vi "Acquisition Message Loop.vi"(8 "error in (no error)":errorcluster, 9 "data queue in":refnum<queue>, 10 "notifier out":refnum<notifier>, 11 "Message Queues":T3) -> (0 "error out":errorcluster)   [LabVIEW 2026, in "Acquisition.lvlib"]
doc: "Message loop for handling messages pertaining to the acquisition of data from the hardware."
uses:
  Acquisition.lvlib
  support/Message Queue/All Message Queues.ctl
  support/Message Queue/Message Cluster.ctl
  controls/NotifierAndDataQueue.ctl
  controls/WaveformChartData.ctl
  Hardware Configuration.ctl
  Acquisition State.ctl
  support/Message Queue/Enqueue Message (Single).vi
  <vilib>/Utility/error.llb/Error Cluster From Error Code.vi
  <vilib>/ErrorRing/Error Ring.xnode
  support/Message Queue/Message Queue.lvlib
  <vilib>/Utility/miscctls.llb/LVRowAndColumnTypeDef.ctl
  Control/Control.lvlib
  Settings/Settings.lvlib
panel:
  out "STOP Button Pressed 4":bool
  out "Pressure Decay Hold Test Complete":bool
  out "STOP Button Pressed 3":bool
  out "Timeout":bool
  out "Pressure Stabilized":bool
  out "STOP Button Pressed 2":bool
  out "Free Air Flow Measurement Complete":bool
  out "RPM Target Reached":bool
  out "STOP Button Pressed":bool
  out "RPM Timeout":bool
  in  "Notifier Data":T1
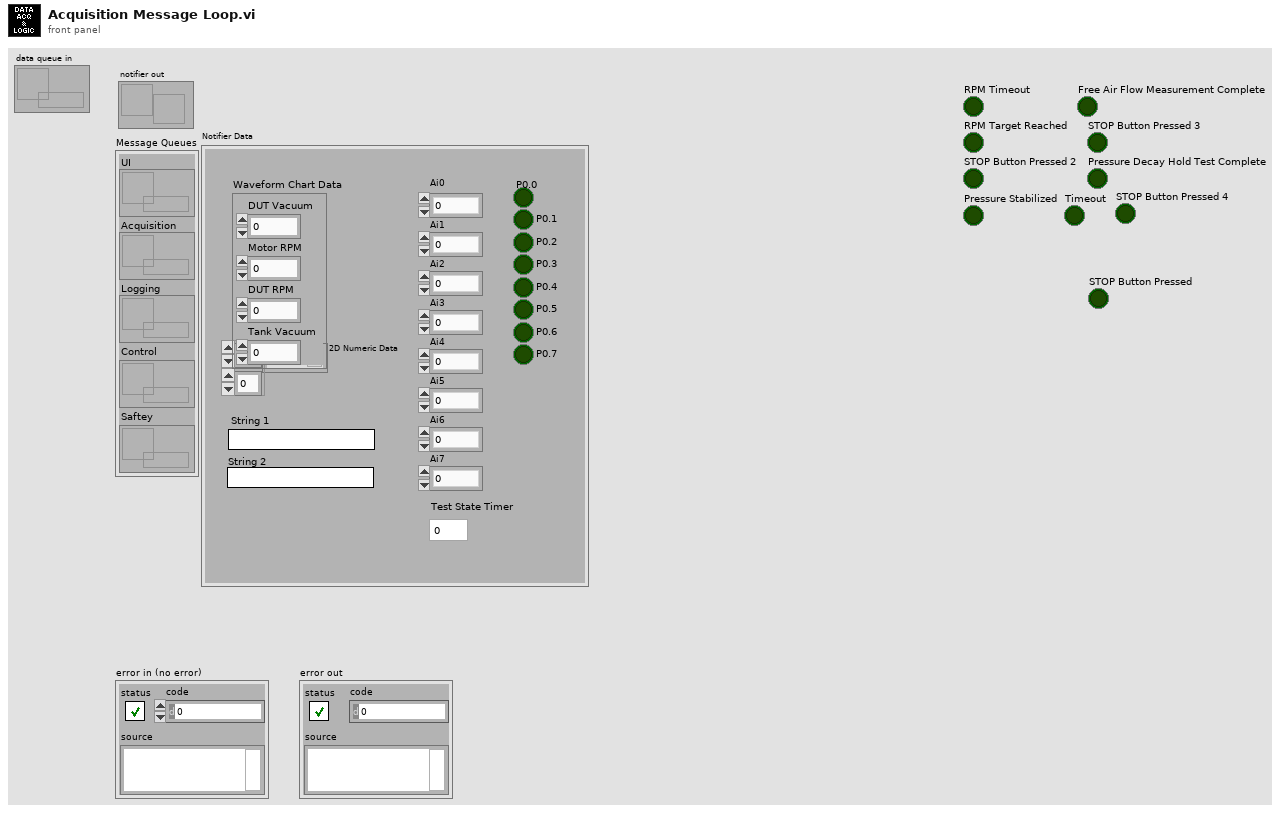
[diagram p1: front panel]
types:
  T1 = typedef "NotifierAndDataQueue.ctl" = cluster{"Ai0":dbl, "Ai1":dbl, "Ai2":dbl, "Ai3":dbl, "Ai4":dbl, "Ai5":dbl, "Ai6":dbl, "Ai7":dbl, "P0.0":bool, "P0.1":bool, "P0.2":bool, "P0.3":bool, "P0.4":bool, "P0.5":bool, "P0.6":bool, "P0.7":bool, "2D Numeric Data":dbl[][], "String 2":string, "String 1":string, "Waveform Chart Data":T2, "Test State Timer":dbl}
  T2 = typedef "Settings.lvlib/WaveformChartData.ctl" = cluster{"DUT Vacuum":dbl, "Motor RPM":dbl, "DUT RPM":dbl, "Tank Vacuum":dbl}
  T3 = typedef "Message Queue.lvlib/All Message Queues.ctl" = cluster{"UI":refnum<queue>, "Acquisition":refnum<queue>, "Logging":refnum<queue>, "Control":refnum<queue>, "Saftey":refnum<queue>}
  T4 = typedef "Acquisition.lvlib/Acquisition State.ctl" = enum16{"Idle", "Acquiring"}
  T5 = typedef "Acquisition.lvlib/Hardware Configuration.ctl" = cluster{"Analog Out array":dbl[], "Initialize Flag":bool, "Saftey Table Display":refnum<vi>, "Torque&Force":waveform(dbl)[][], "Calibration Data":waveform(dbl)[], "2D":dbl[][], "Analog In Task":refnum<k21>, "Digital In Task":refnum<k21>, "Analog Out Task":refnum<k21>, "Digital Out Task":refnum<k21>, "Digital Out Array":bool[], "Current Cycle Count":refnum<vi>, "Cycle Count":u64, "Headers":string[], "Sweep Interval":u64, "Delay":u64, "TestConfigDisplay":refnum<vi>, "50psi Conversion":dbl[], "1245N15 Conversion":dbl[], "MX06F Conversion":dbl[], "# of Test Cycles":u64, "60psi Conversion":dbl[], "100psi Conversion":dbl[], "200psi Conversion":dbl[], "1000psi Conversion":dbl[], "2000psi Conversion":dbl[], "5000psi Conversion":dbl[], "MX09F Conversion":dbl[], "MX19F Conversion":dbl[], "DUT VALVE POSITION":refnum<vi>, "INTAKE VALVE POSITION":refnum<vi>, "Table Control":refnum<vi>, "Table Control":string[][], "Max Vacuum":dbl, "RPM Ramp Ref":refnum<vi>, "Free Air Flow Ref":refnum<vi>, "Press Stable Ref":refnum<vi>, "Press Decay Ref":refnum<vi>}
  T6 = typedef "LVRowAndColumnTypeDef.ctl" = cluster{"Row":i32, "Column":i32}
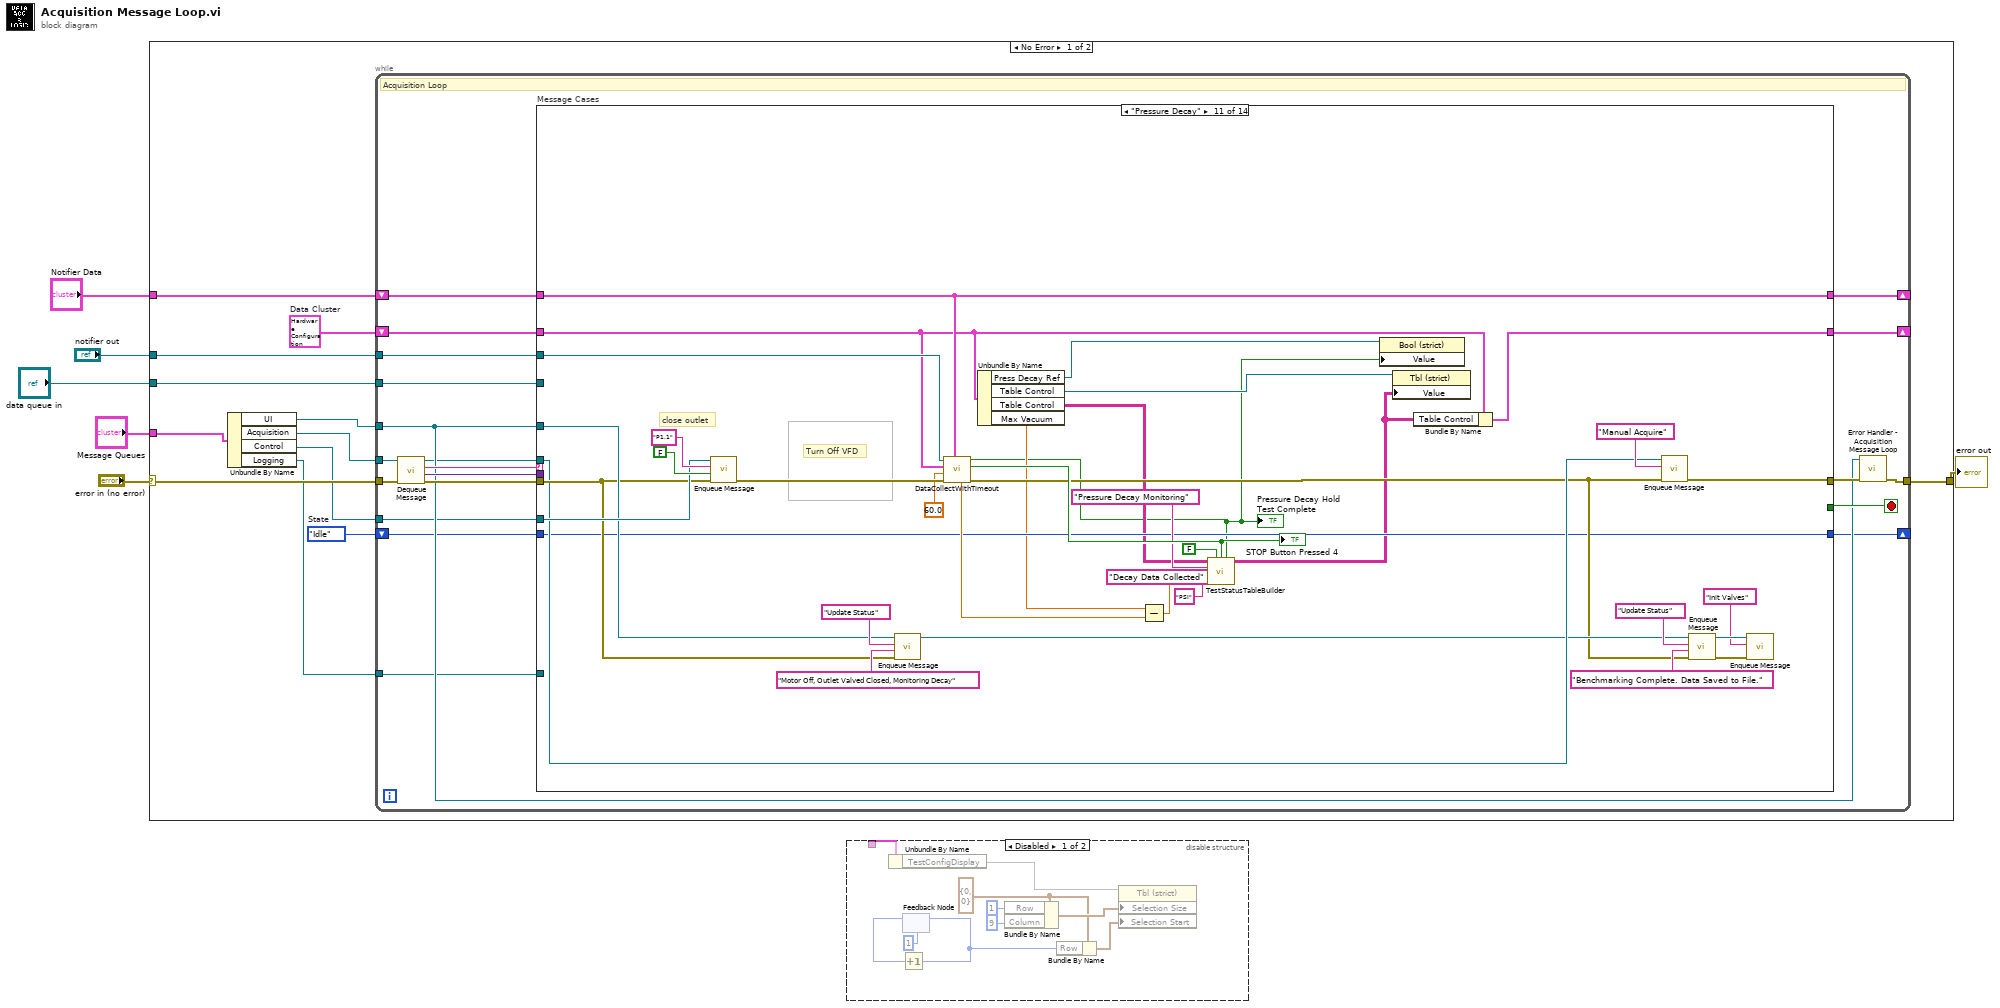
[diagram p0: block diagram]
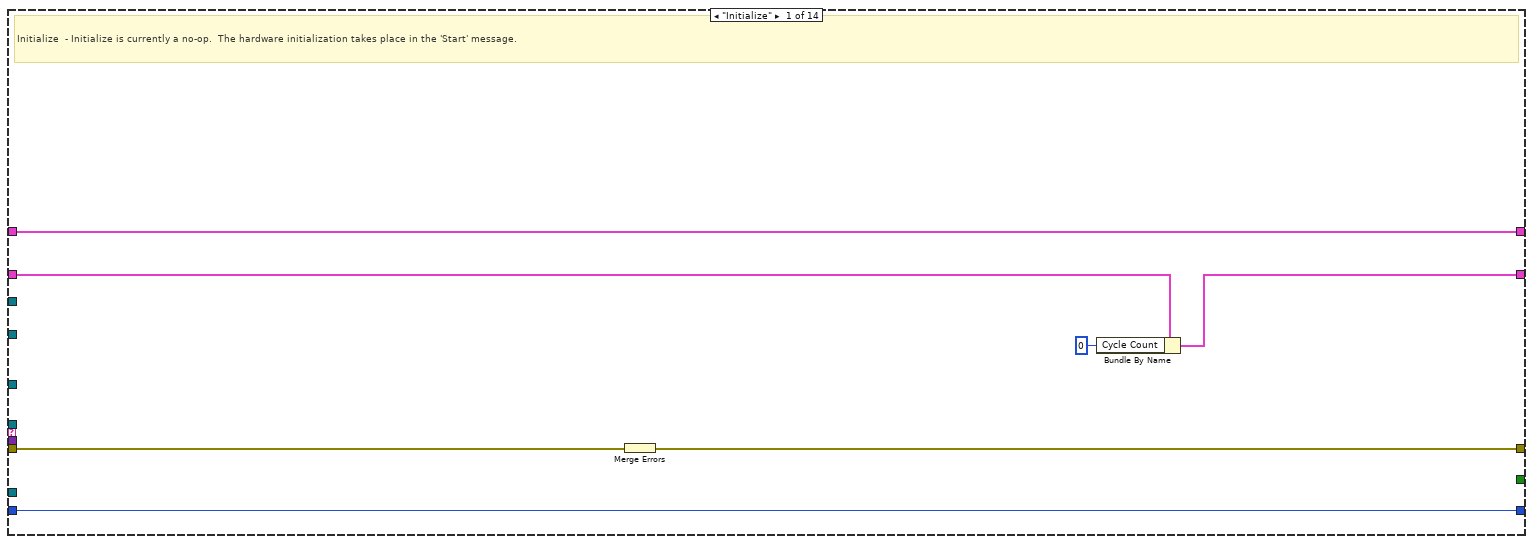
[diagram p3: hidden frame]
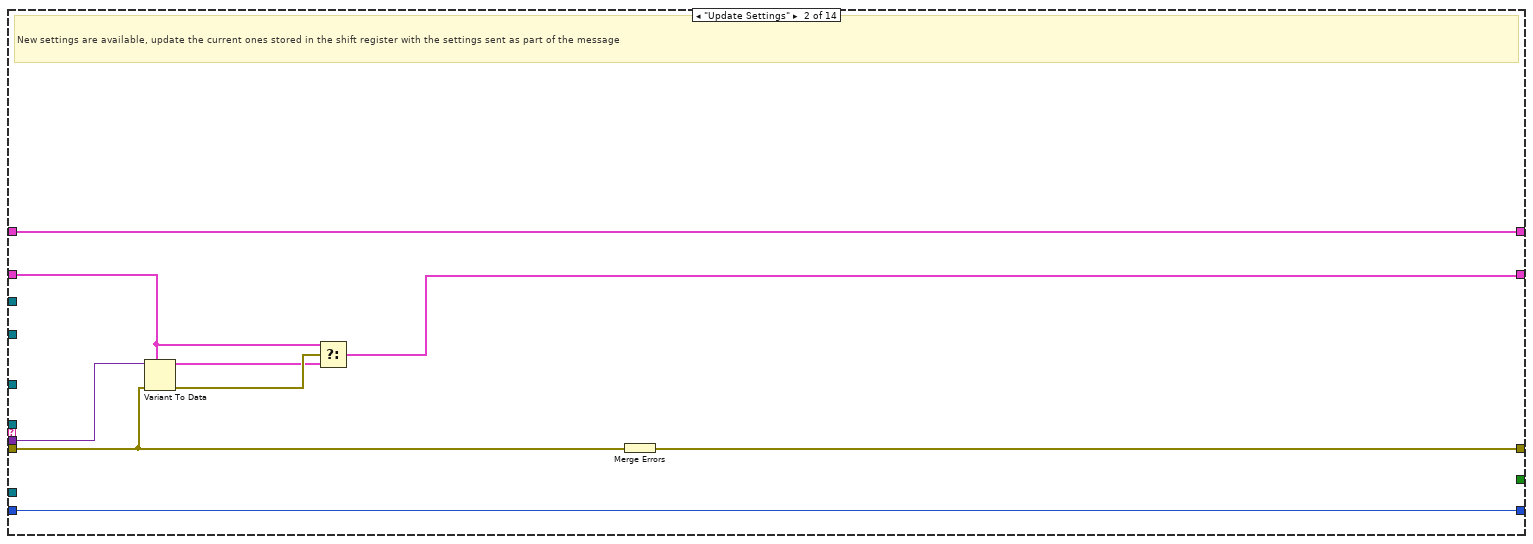
[diagram p4: hidden frame]
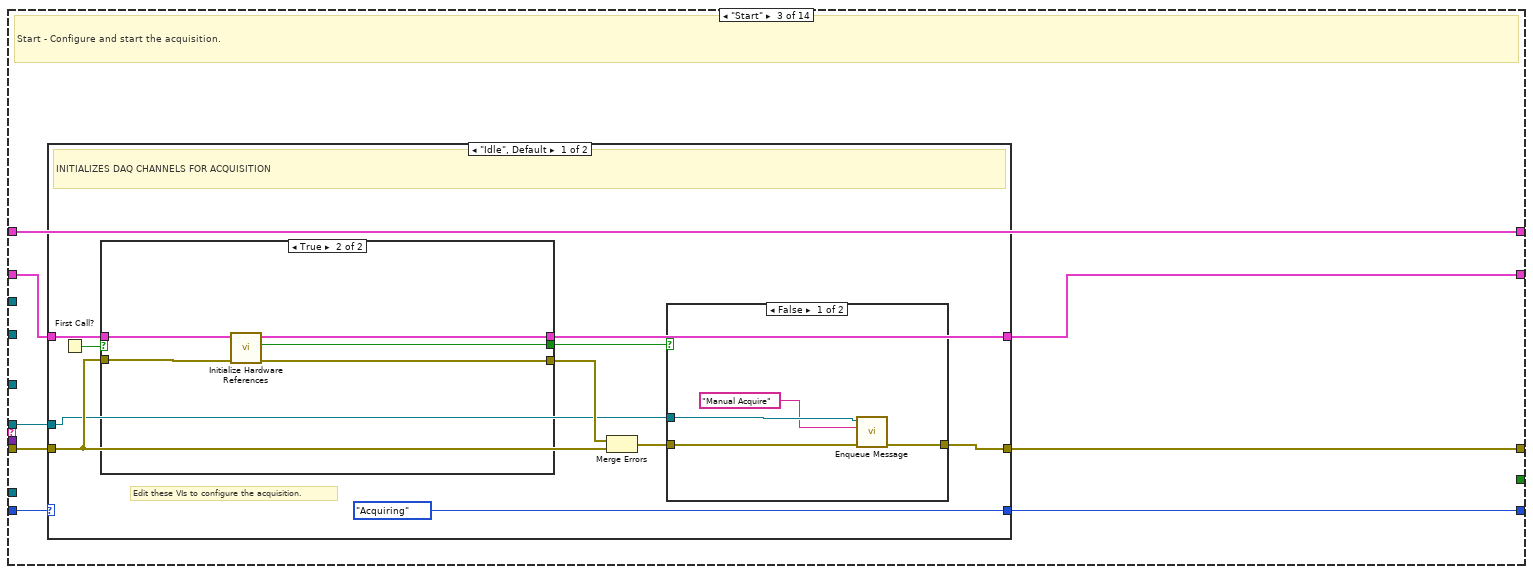
[diagram p5: hidden frame]
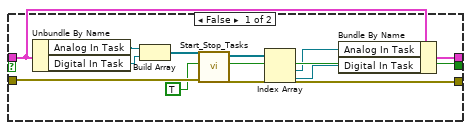
[diagram p6: hidden frame]
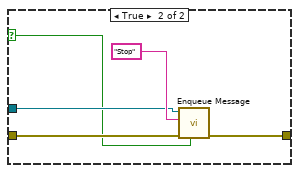
[diagram p7: hidden frame]
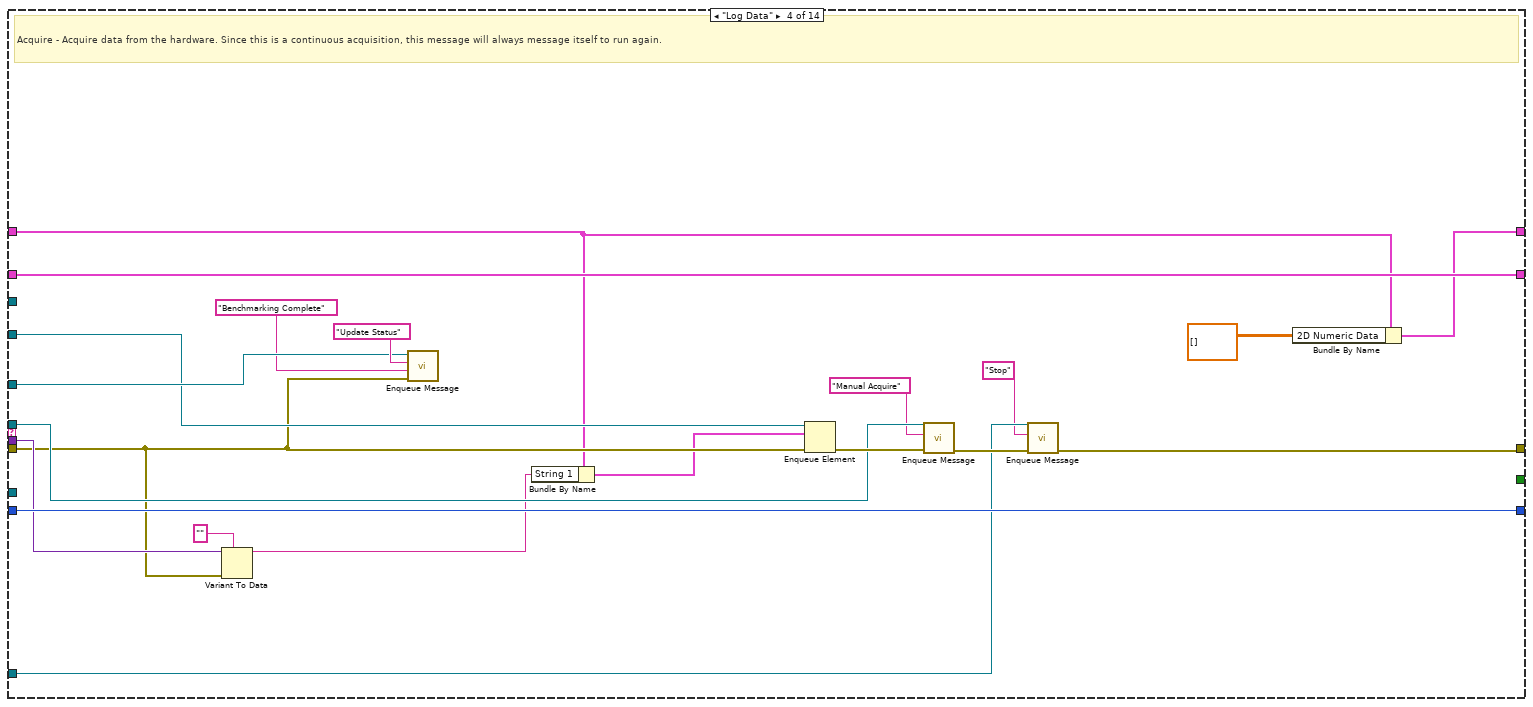
[diagram p9: hidden frame]
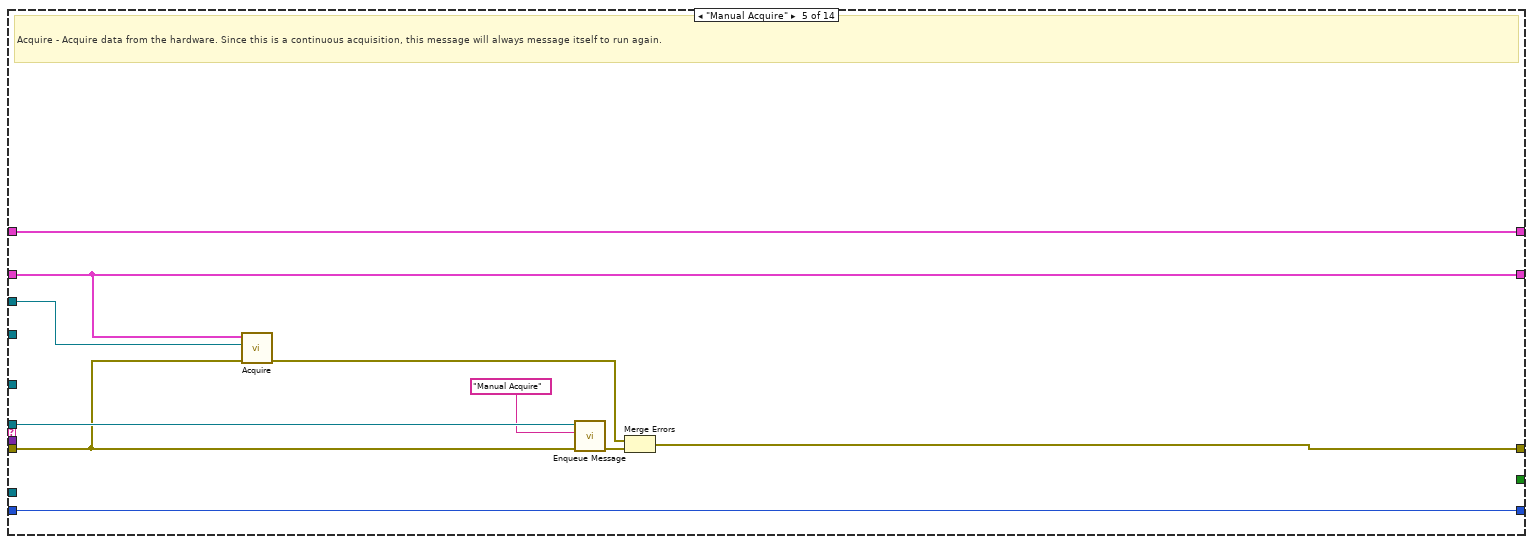
[diagram p10: hidden frame]
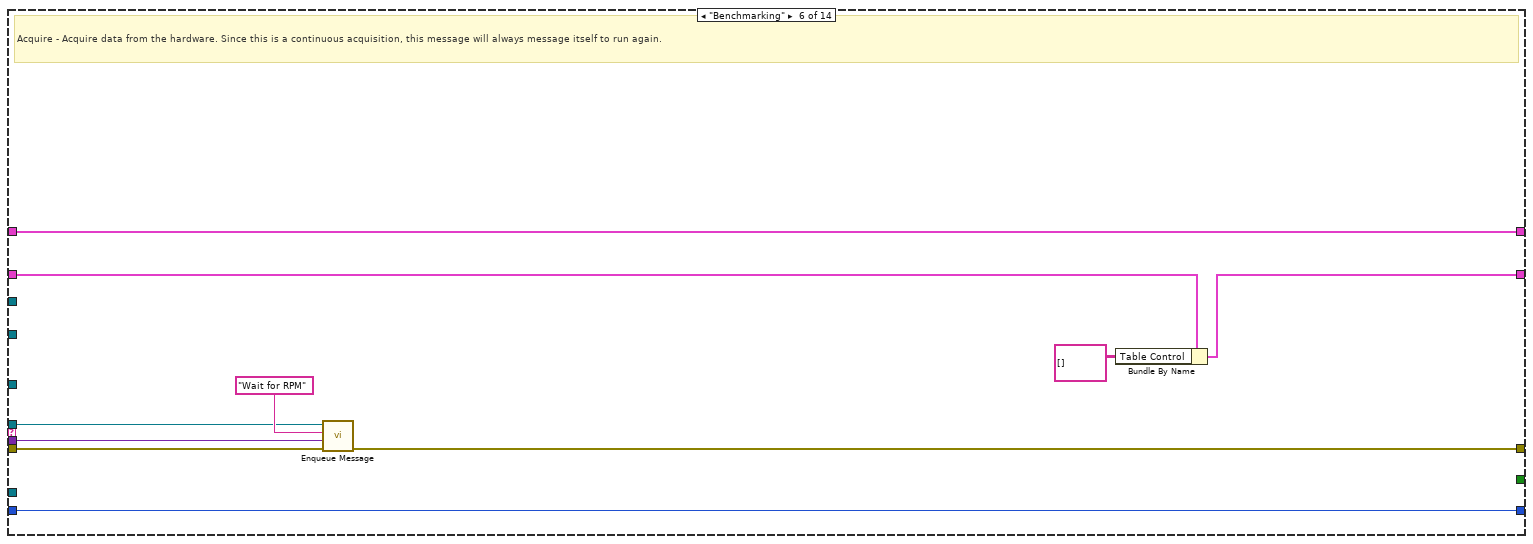
[diagram p11: hidden frame]
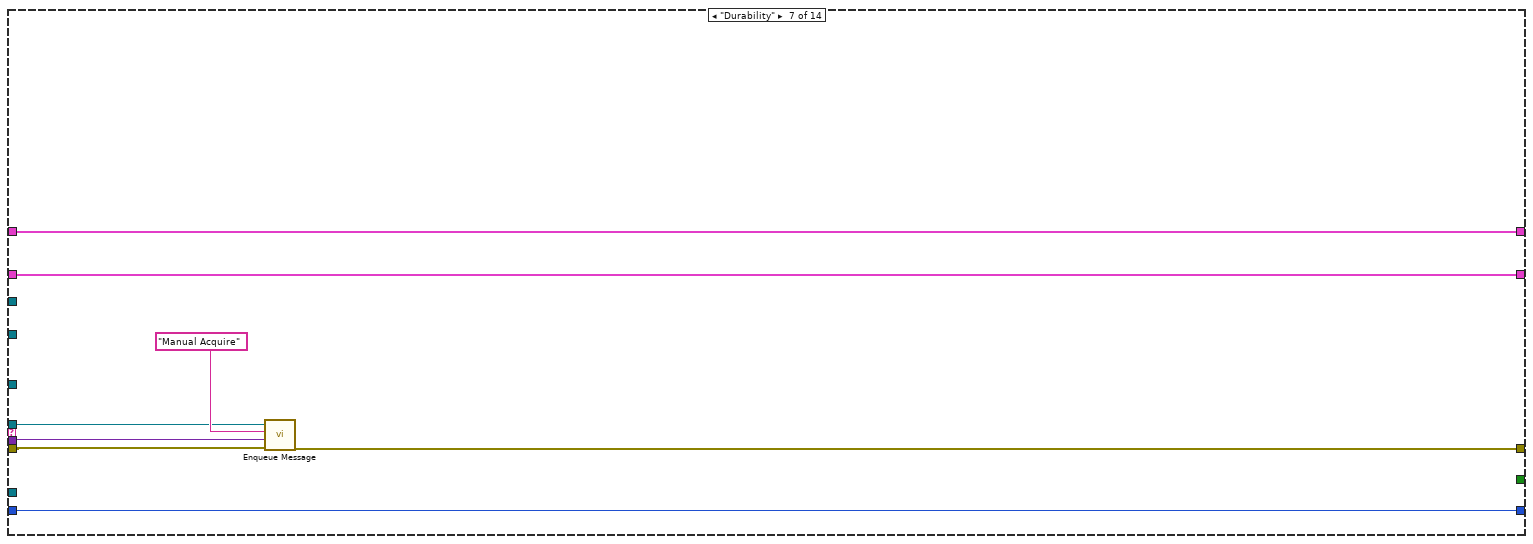
[diagram p12: hidden frame]
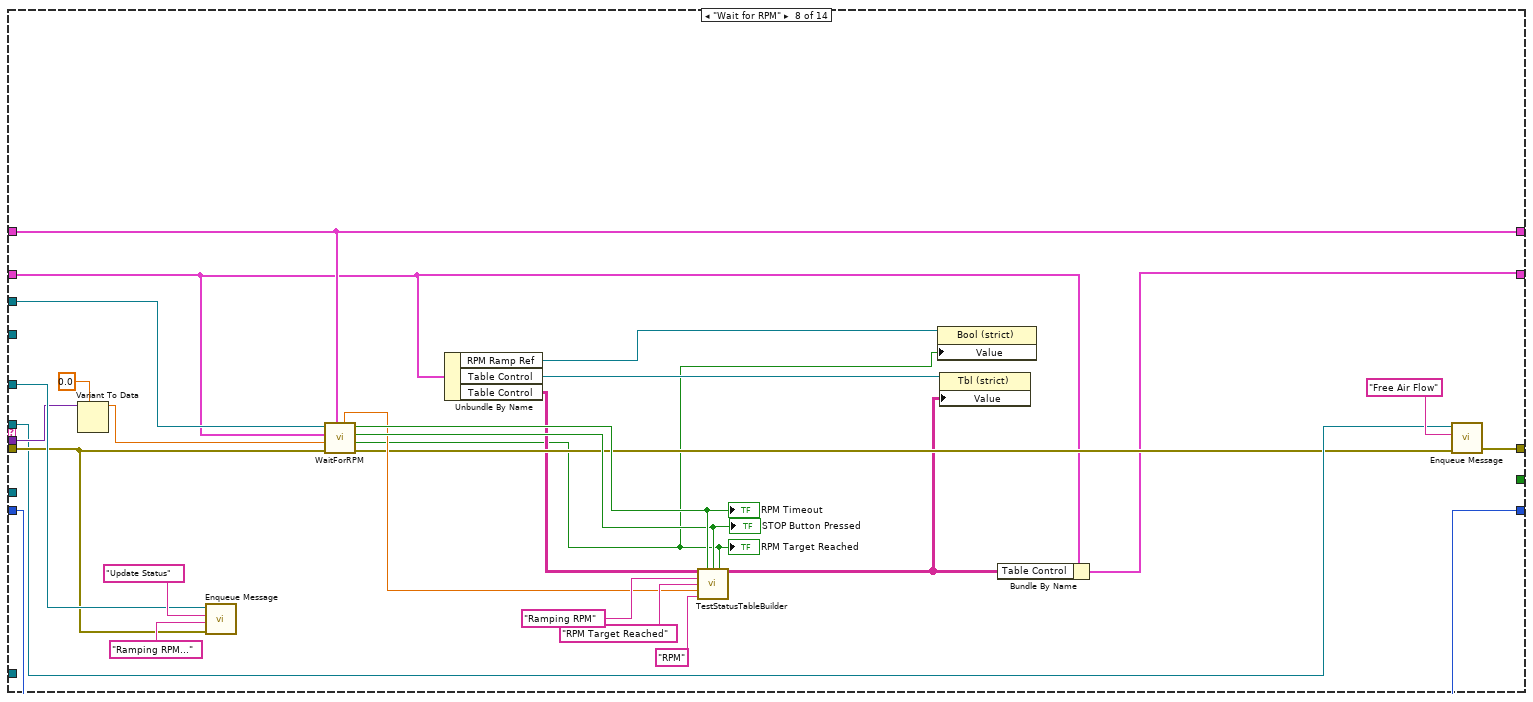
[diagram p13: hidden frame]
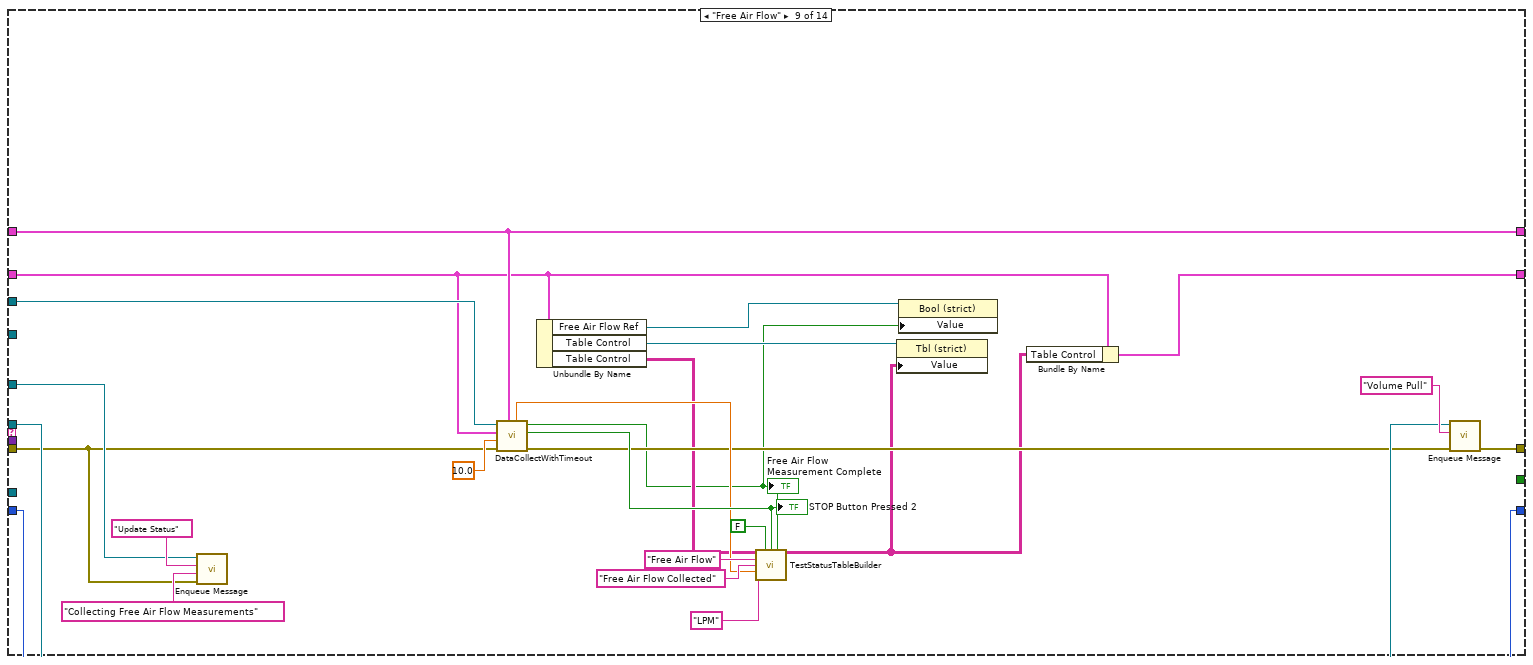
[diagram p14: hidden frame]
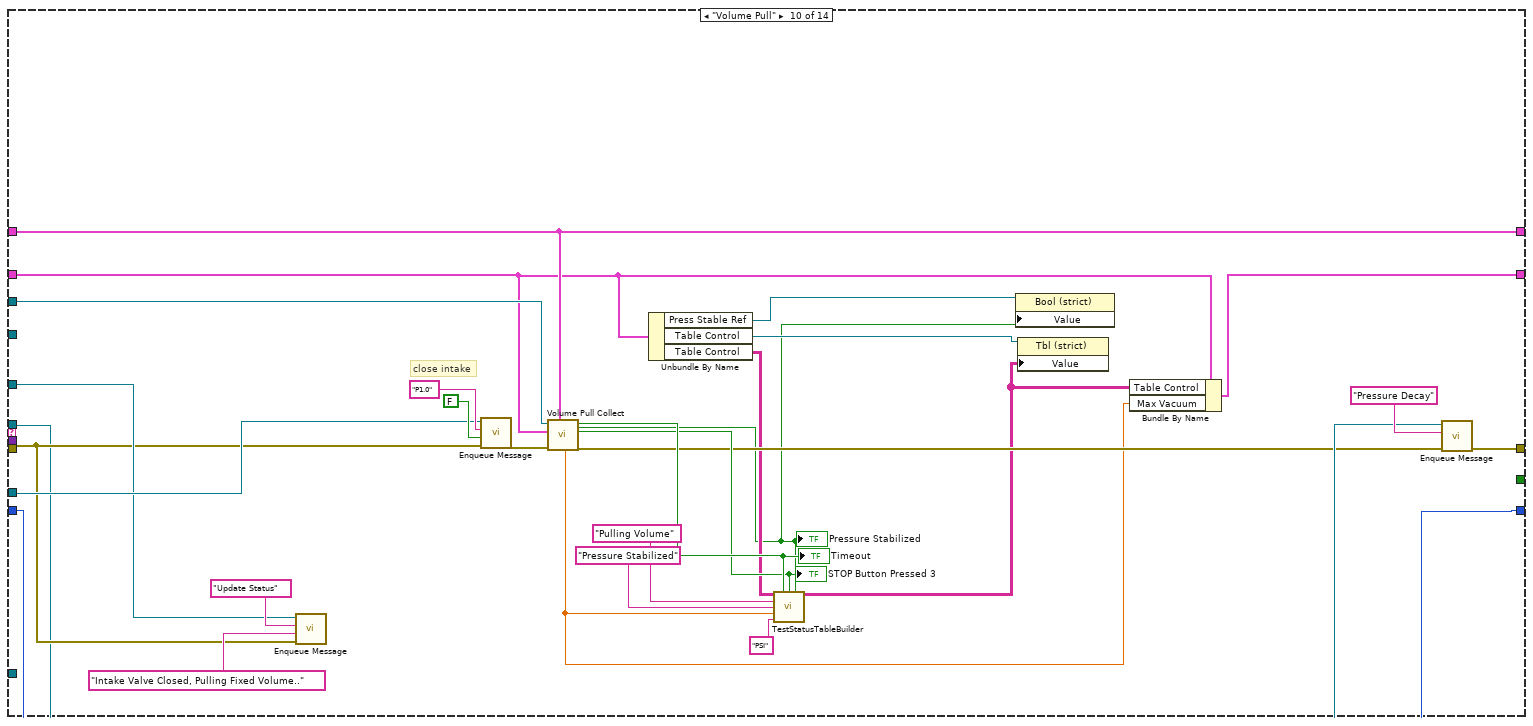
[diagram p15: hidden frame]
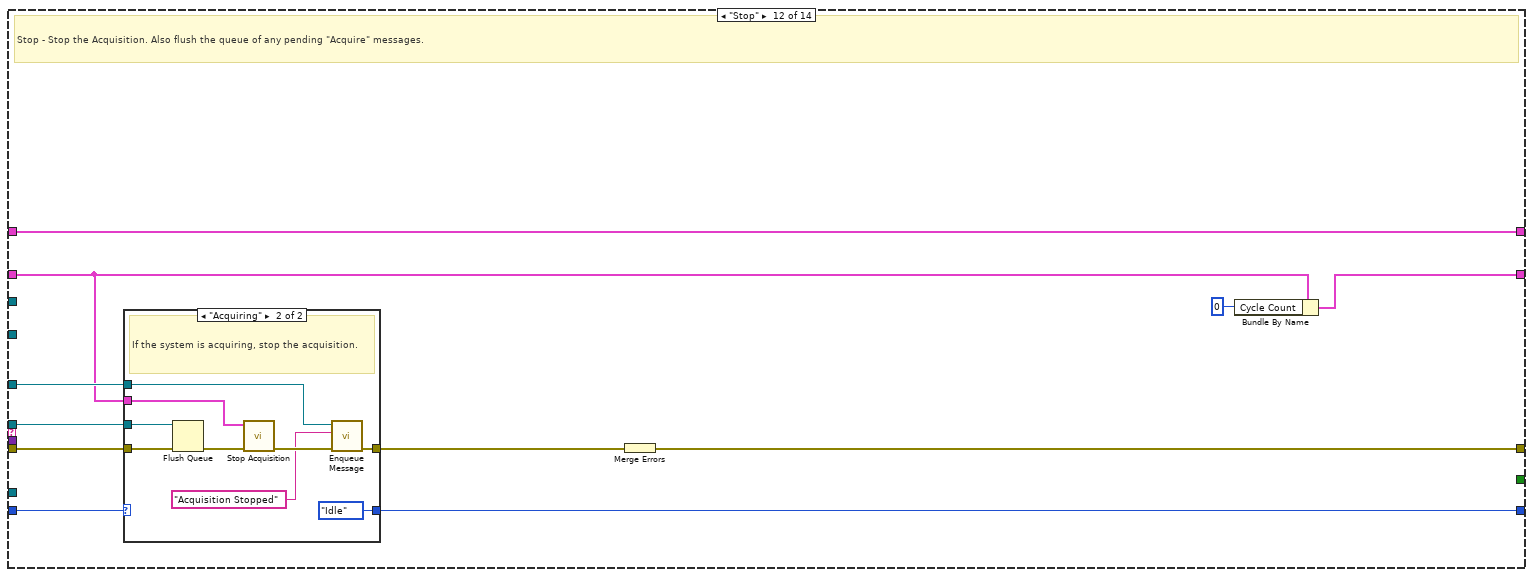
[diagram p16: hidden frame]
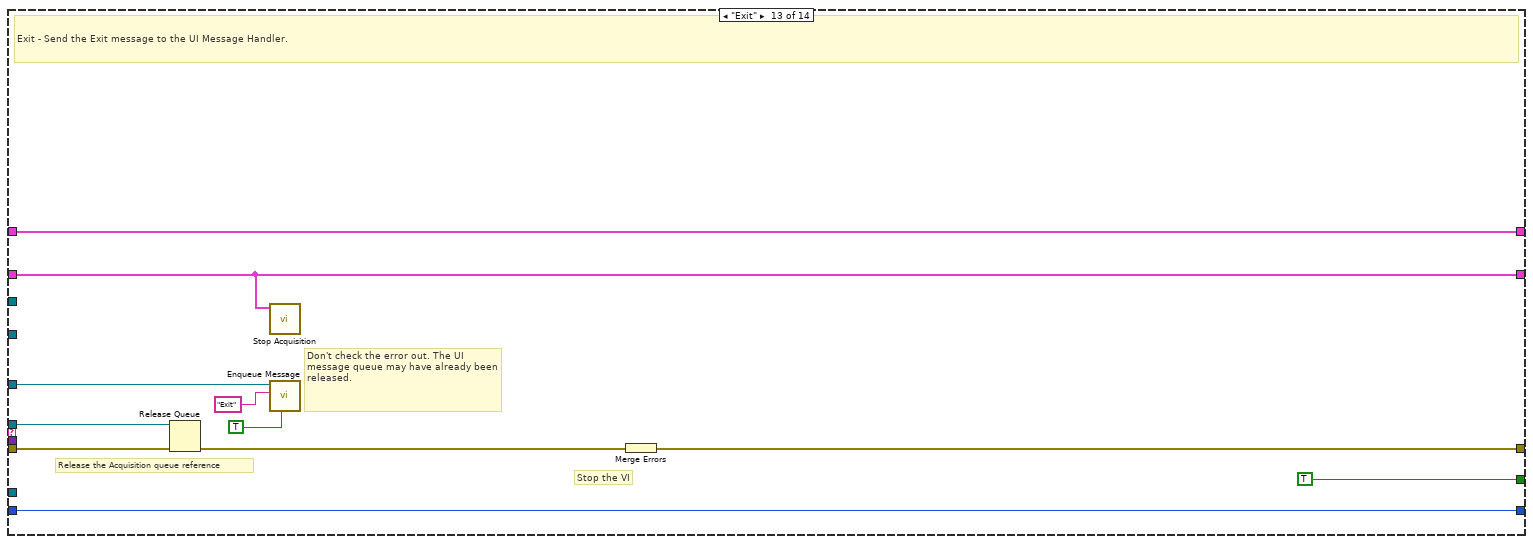
[diagram p18: hidden frame]
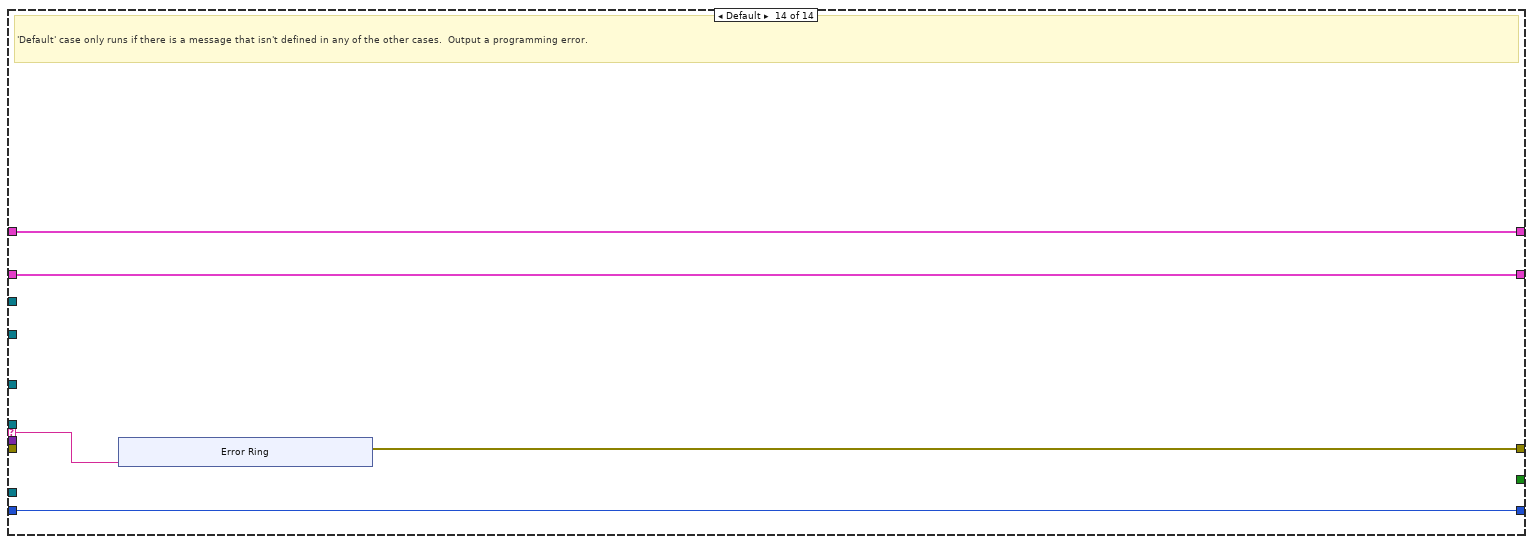
[diagram p19: hidden frame]
diagram:
  n1 = case shown="No Error" "error in (no error)" {
    selector: "error in (no error)" -> [w14 w313]
    tunnel: "Message Queues" -> [w18 _]
    tunnel: [w16 w313] -> w5
    tunnel: "notifier out" -> [w12 _]
    tunnel: "data queue in" -> [w11 _]
    tunnel: "Notifier Data" -> [w8 _]
    frame No Error {
      w10 = Acquisition_State."Idle"  # State
      w15 = T5 {"Analog Out array"=[], "Initialize Flag"=FALSE, "Saftey Table Display"=refnum, "Torque&Force"=[], "Calibration Data"=[], "2D"=[], "Analog In Task"="", "Digital In Task"="", "Analog Out Task"="", "Digital Out Task"="", "Digital Out Array"=[], "Current Cycle Count"=refnum, "Cycle Count"=0, "Headers"=[], "Sweep Interval"=0, "Delay"=0, "TestConfigDisplay"=refnum, "50psi Conversion"=[], "1245N15 Conversion"=[], "MX06F Conversion"=[], "# of Test Cycles"=0, "60psi Conversion"=[], "100psi Conversion"=[], "200psi Conversion"=[], "1000psi Conversion"=[], "2000psi Conversion"=[], "5000psi Conversion"=[], "MX09F Conversion"=[], "MX19F Conversion"=[], "DUT VALVE POSITION"=refnum, "INTAKE VALVE POSITION"=refnum, "Table Control"=refnum, "Table Control"=[], "Max Vacuum"=0.0, "RPM Ramp Ref"=refnum, "Free Air Flow Ref"=refnum, "Press Stable Ref"=refnum, "Press Decay Ref"=refnum}  # Data Cluster
      n2 = Unbundle By Name(w18) -> ("UI"=w13:refnum<queue>, "Acquisition"=w17:refnum<queue>, "Control"=w9:refnum<queue>, "Logging"=w7:refnum<queue>)
      n3 = while {
        tunnel: w17 -> [w23]
        shift-right: [w37] -> _
        shift-left: w15 -> [w38]
        tunnel: w13 -> [w27]
        tunnel: w12 -> [w31]
        tunnel: w11 -> [w30]
        shift-right: [w25] -> _
        shift-left: w10 -> [w26]
        tunnel: w9 -> [w24]
        tunnel: w14 -> [w35]
        tunnel: [w28] -> w16
        shift-right: [w20] -> _
        shift-left: w8 -> [w21]
        tunnel: w7 -> [w19]
        stop <- w36 stop-if-true
        # "Acquisition Loop"
        n4 = call "Dequeue Message.vi"("error in (no error)"=w35, "Message Queue"=w23) -> ("error out"=w34:errorcluster, "Message Data"=w32:variant, "Message"=w33:string, "dup Message Queue"=w22:refnum<queue>)  [unwired: 6 in]
        n5 = case "Message Cases" shown="\"Pressure Decay\"" w33 {
          selector: w33 -> [_ _ _ _ _ _ _ _ _ _ _ _ _ w304]
          tunnel: w22 -> [_ _ w60 w113 w130 w141 w148 w159 w190 w212 w243 w276 w293 _]
          tunnel: w34 -> [w44 w48 w61 w110 w129 w139 w147 w168 w189 w218 w251 w277 w297 _]
          tunnel: [w45 w54 w56 w102 w132 w140 w145 w160 w192 w213 w244 w278 w299 w303] -> w29
          tunnel: w38 -> [w41 w50 w62 w117 w123 w135 w150 w156 w183 w209 w237 w269 w292 w305]
          tunnel: [w40 w49 w59 w117 w123 w134 w150 w155 w182 w208 w236 w268 w292 w305] -> w37
          tunnel: [_ _ _ _ _ _ _ _ _ _ _ _ TRUE _] -> w36
          tunnel: w32 -> [_ w53 _ w111 _ w138 w146 w165 _ _ _ _ _ _]
          tunnel: w27 -> [_ _ _ w120 _ _ _ w169 w193 w219 w252 w275 w298 _]
          tunnel: w31 -> [_ _ _ _ w126 _ _ w167 w187 w217 w253 _ _ _]
          tunnel: w30 -> [_ _ _ w118 _ _ _ _ _ _ _ _ _ _]
          tunnel: w26 -> [w43 w47 w58 w122 w125 w137 w144 w162 w185 w216 w240 w274 w291 w302]
          tunnel: [w43 w47 w57 w122 w125 w137 w144 w162 w185 w216 w240 w273 w291 w302] -> w25
          tunnel: w24 -> [_ _ _ _ _ _ _ _ _ w220 w254 _ _ _]
          tunnel: w21 -> [w42 w46 w55 w108 w124 w136 w143 w166 w186 w215 w239 w270 w290 w301]
          tunnel: [w42 w46 w55 w116 w124 w136 w143 w166 w186 w215 w239 w270 w290 w301] -> w20
          tunnel: w19 -> [_ _ _ w104 _ _ _ _ _ _ _ _ _ _]
          frame "Initialize" {
            # "Initialize  - Initialize is currently a no-op.  The hardware initialization takes place in the 'Start' message."
            n6 = Merge Errors(w44) -> (w45:errorcluster)
            n7 = Bundle By Name(cluster=w41, "Cycle Count"=u64 0) -> (w40:T5)
          }
          frame "Update Settings" {
            # "New settings are available, update the current ones stored in the shift register with the settings sent as part of the message"
            n8 = Variant To Data(error in=w48, type=w50, Variant=w53) -> (data=w51:T5, error out=w52:errorcluster)
            n9 = Select(t=w50, s=w52, f=w51) -> (s? t:f=w49:T5)
            n10 = Merge Errors(w48) -> (w54:errorcluster)
          }
          frame "Start" {
            # "Start - Configure and start the acquisition."
            n11 = case shown="\"Idle\", Default" w58 {
              selector: w58 -> [_ w99]
              tunnel: [w66 w101] -> w56
              tunnel: w62 -> [w72 w100]
              tunnel: w61 -> [w70 w101]
              tunnel: w60 -> [w64 _]
              tunnel: [w69 w100] -> w59
              tunnel: [Acquisition_State."Acquiring" ("State") w99] -> w57
              frame "Idle", Default {
                # "Edit these VIs to configure the acquisition."
                # "INITIALIZES DAQ CHANNELS FOR ACQUISITION"
                n12 = First Call?() -> (First Call?: T/F=w63:bool)
                n13 = case shown="True" w63 {
                  tunnel: w72 -> [w76 w89]
                  tunnel: w70 -> [w83 w88]
                  tunnel: [w77 w87] -> w69
                  tunnel: [w84 w86] -> w68
                  tunnel: [w82 w85] -> w65
                  frame False {
                    n14 = Unbundle By Name(w76) -> ("Analog In Task"=w80:refnum<k21>, "Digital In Task"=w79:refnum<k21>)
                    n15 = Build Array(w80, w79) -> (w78:refnum<k21>[])
                    n16 = call "Start_Stop_Tasks.vi"("error in"=w83, "Start/Stop Task"=TRUE, "Tasks In"=w78) -> ("error out"=w84:errorcluster, "error?"=w82:bool, "Tasks Out"=w75:refnum<k21>[])  [unwired: 6 in]
                    n17 = Index Array(array=w75) -> (element #1=w74:refnum<k21>, element #2=w73:refnum<k21>)  [unwired: 2 in]
                    n18 = Bundle By Name(cluster=w76, "Analog In Task"=w74, "Digital In Task"=w73) -> (w77:T5)
                  }
                  frame True {
                    n19 = call "Initialize Hardware References.vi"("error in (no error)"=w88, "Hardware Resources in"=w89) -> ("error out"=w86:errorcluster, "error?"=w85:bool, "Hardware Resources out"=w87:T5)  [unwired: 7 in]
                  }
                }
                n20 = Merge Errors(w68, w70) -> (w67:errorcluster)
                n21 = case shown="False" w65 {
                  selector: w65 -> [_ w94]
                  tunnel: w67 -> [w93 w97]
                  tunnel: [w91 w96] -> w66
                  tunnel: w64 -> [w92 w95]
                  frame False {
                    n22 = call-poly "Enqueue Message.vi"("error in (no error)"=w93, "Message"="Manual Acquire", "Message Queue"=w92) -> ("error out"=w91:errorcluster)  [unwired: 7 in, 1 out]
                  }
                  frame True {
                    n23 = call-poly "Enqueue Message.vi"("Priority Message? (F)"=w94, "error in (no error)"=w97, "Message"="Stop", "Message Queue"=w95) -> ("error out"=w96:errorcluster)  [unwired: 6 in, 1 out]
                  }
                }
              }
              frame "Acquiring" {
                # "The system is already acquiring. Ignore the \"Start\" message."
              }
            }
          }
          frame "Log Data" {
            # "Acquire - Acquire data from the hardware. Since this is a continuous acquisition, this message will always message itself to run again."
            n24 = Variant To Data(error in=w110, type="", Variant=w111) -> (data=w107:string)  [unwired: 1 out]
            n25 = call-poly "Enqueue Message.vi"("error in (no error)"=w110, "Message Data"="Benchmarking Complete" ("Message"), "Message"="Update Status", "Message Queue"=w120) -> ()  [unwired: 6 in, 2 out]
            n26 = Bundle By Name(cluster=w108, "String 1"=w107) -> (w106:T1)
            n27 = Enqueue Element(queue=w118, element=w106, error in (no error)=w110) -> (error out=w114:errorcluster)  [unwired: 1 in, 2 out]
            n28 = call-poly "Enqueue Message.vi"("error in (no error)"=w114, "Message"="Manual Acquire", "Message Queue"=w113) -> ("error out"=w105:errorcluster)  [unwired: 7 in, 1 out]
            n29 = call-poly "Enqueue Message.vi"("error in (no error)"=w105, "Message"="Stop", "Message Queue"=w104) -> ("error out"=w102:errorcluster)  [unwired: 7 in, 1 out]
            n30 = Bundle By Name(cluster=w108, "2D Numeric Data"=dbl[][] [] ("Torqe & force 2D")) -> (w116:T1)
          }
          frame "Manual Acquire" {
            # "Acquire - Acquire data from the hardware. Since this is a continuous acquisition, this message will always message itself to run again."
            n31 = call "Acquire.vi"("error in (no error)"=w129, "notifier out"=w126, "Hardware Resources in"=w123) -> ("error out"=w128:errorcluster)  [unwired: 6 in, 2 out]
            n32 = call-poly "Enqueue Message.vi"("error in (no error)"=w129, "Message"="Manual Acquire", "Message Queue"=w130) -> ("error out"=w131:errorcluster)  [unwired: 7 in, 1 out]
            n33 = Merge Errors(w128, w131) -> (w132:errorcluster)
          }
          frame "Benchmarking" {
            # "Acquire - Acquire data from the hardware. Since this is a continuous acquisition, this message will always message itself to run again."
            n34 = call-poly "Enqueue Message.vi"("error in (no error)"=w139, "Message Data"=w138, "Message"="Wait for RPM", "Message Queue"=w141) -> ("error out"=w140:errorcluster)  [unwired: 6 in, 1 out]
            n35 = Bundle By Name(cluster=w135, "Table Control"=string[][] []) -> (w134:T5)
          }
          frame "Durability" {
            n36 = call-poly "Enqueue Message.vi"("error in (no error)"=w147, "Message Data"=w146, "Message"="Manual Acquire", "Message Queue"=w148) -> ("error out"=w145:errorcluster)  [unwired: 6 in, 1 out]
          }
          frame "Wait for RPM" {
            n37 = Variant To Data(type=0.0, Variant=w165) -> (data=w163:dbl)  [unwired: 1 in, 1 out]
            n38 = call-poly "Enqueue Message.vi"("error in (no error)"=w168, "Message Data"="Ramping RPM..." ("Message"), "Message"="Update Status", "Message Queue"=w169) -> ()  [unwired: 6 in, 2 out]
            n39 = call "WaitForRPM.vi"("Notifier Data"=w166, "error in (no error)"=w168, "RPM target"=w163, "Data Cluster"=w156, "Notifier in"=w167) -> ("error out"=w158:errorcluster, "RPM Target Reached"=w151:bool, "STOP Button Pressed"=w174:bool, "RPM Timeout"=w175:bool, "RPM"=w170:dbl)  [unwired: 2 in]
            "RPM Timeout" <- w175
            "STOP Button Pressed" <- w174
            "RPM Target Reached" <- w151
            n40 = Unbundle By Name(w156) -> ("RPM Ramp Ref"=w152:refnum<vi>, "Table Control"=w154:refnum<vi>, "Table Control"=w157:string[][])
            n41 = call "TestStatusTableBuilder.vi"("array"=w157, "Test Case Timeout"=w175, "STOP Button Pressed"=w174, "Test Case Target Reached"=w151, "Test State"="Ramping RPM", "Test Status"="RPM Target Reached", "Measurement"=w170, "Units"="RPM") -> ("Table Control"=w153:string[][])  [unwired: 7 in]
            n42 = property class="Bool (strict)"(reference=w152, "Value"=w151) -> ()  [unwired: 1 in, 2 out]
            n43 = property class="Tbl (strict)"(reference=w154, "Value"=w153) -> ()  [unwired: 1 in, 2 out]
            n44 = Bundle By Name(cluster=w156, "Table Control"=w153) -> (w155:T5)
            n45 = call-poly "Enqueue Message.vi"("error in (no error)"=w158, "Message"="Free Air Flow", "Message Queue"=w159) -> ("error out"=w160:errorcluster)  [unwired: 7 in, 1 out]
          }
          frame "Free Air Flow" {
            n46 = call-poly "Enqueue Message.vi"("error in (no error)"=w189, "Message Data"="Collecting Free Air Flow Measurements" ("Message"), "Message"="Update Status", "Message Queue"=w193) -> ()  [unwired: 6 in, 2 out]
            n47 = call "DataCollectWithTimeout.vi"("Notifier Data"=w186, "error in (no error)"=w189, "Timeout"=10.0, "Data Cluster"=w183, "Notifier in"=w187) -> ("error out"=w188:errorcluster, "STOP Button Pressed"=w201:bool, "Free Air Flow Measurement Complete"=w178:bool, "Air Flow Data"=w196:dbl)  [unwired: 1 in, 2 out]
            "Free Air Flow Measurement Complete" <- w178
            "STOP Button Pressed 2" <- w201
            n48 = Unbundle By Name(w183) -> ("Free Air Flow Ref"=w179:refnum<vi>, "Table Control"=w180:refnum<vi>, "Table Control"=w184:string[][])
            n49 = call "TestStatusTableBuilder.vi"("array"=w184, "Test Case Timeout"=FALSE, "STOP Button Pressed"=w201, "Test Case Target Reached"=w178, "Test State"="Free Air Flow", "Test Status"="Free Air Flow Collected", "Measurement"=w196, "Units"="LPM") -> ("Table Control"=w181:string[][])  [unwired: 7 in]
            n50 = property class="Tbl (strict)"(reference=w180, "Value"=w181) -> ()  [unwired: 1 in, 2 out]
            n51 = property class="Bool (strict)"(reference=w179, "Value"=w178) -> ()  [unwired: 1 in, 2 out]
            n52 = Bundle By Name(cluster=w183, "Table Control"=w181) -> (w182:T5)
            n53 = call-poly "Enqueue Message.vi"("error in (no error)"=w188, "Message"="Volume Pull", "Message Queue"=w190) -> ("error out"=w192:errorcluster)  [unwired: 7 in, 1 out]
          }
          frame "Volume Pull" {
            # "close intake"
            n54 = call-poly "Enqueue Message.vi"("error in (no error)"=w218, "Message Data"="Intake Valve Closed, Pulling Fixed Volume.." ("Message"), "Message"="Update Status", "Message Queue"=w219) -> ()  [unwired: 6 in, 2 out]
            n55 = call-poly "Enqueue Message.vi"("error in (no error)"=w218, "Message Data"=FALSE, "Message"="P1.0", "Message Queue"=w220) -> ("error out"=w228:errorcluster)  [unwired: 6 in, 1 out]
            n56 = call "Volume Pull Collect.vi"("Notifier Data"=w215, "error in (no error)"=w228, "Data Cluster"=w209, "Notifier in"=w217) -> ("error out"=w211:errorcluster, "STOP Button Pressed"=w224:bool, "Timeout"=w225:bool, "Stabilzed Pressure"=w205:dbl, "Pressure Stabilized"=w203:bool)  [unwired: 2 in, 1 out]
            "Pressure Stabilized" <- w203
            "Timeout" <- w225
            "STOP Button Pressed 3" <- w224
            n57 = Unbundle By Name(w209) -> ("Press Stable Ref"=w204:refnum<vi>, "Table Control"=w206:refnum<vi>, "Table Control"=w210:string[][])
            n58 = call "TestStatusTableBuilder.vi"("array"=w210, "Test Case Timeout"=w225, "STOP Button Pressed"=w224, "Test Case Target Reached"=w203, "Test State"="Pulling Volume", "Test Status"="Pressure Stabilized", "Measurement"=w205, "Units"="PSI") -> ("Table Control"=w207:string[][])  [unwired: 7 in]
            n59 = property class="Bool (strict)"(reference=w204, "Value"=w203) -> ()  [unwired: 1 in, 2 out]
            n60 = property class="Tbl (strict)"(reference=w206, "Value"=w207) -> ()  [unwired: 1 in, 2 out]
            n61 = Bundle By Name(cluster=w209, "Table Control"=w207, "Max Vacuum"=w205) -> (w208:T5)
            n62 = call-poly "Enqueue Message.vi"("error in (no error)"=w211, "Message"="Pressure Decay", "Message Queue"=w212) -> ("error out"=w213:errorcluster)  [unwired: 7 in, 1 out]
          }
          frame "Pressure Decay" {
            # "Turn Off VFD"
            # "close outlet"
            n63 = call-poly "Enqueue Message.vi"("error in (no error)"=w251, "Message Data"=FALSE, "Message"="P1.1", "Message Queue"=w254) -> ("error out"=w265:errorcluster)  [unwired: 6 in, 1 out]
            n64 = call-poly "Enqueue Message.vi"("error in (no error)"=w251, "Message Data"="Motor Off, Outlet Valved Closed, Monitoring Decay" ("Message"), "Message"="Update Status", "Message Queue"=w252) -> ("dup Message Queue"=w242:refnum<queue>)  [unwired: 6 in, 1 out]
            n65 = call "DataCollectWithTimeout.vi"("Notifier Data"=w239, "error in (no error)"=w265, "Timeout"=60.0, "Data Cluster"=w237, "Notifier in"=w253) -> ("error out"=w241:errorcluster, "STOP Button Pressed"=w260:bool, "Free Air Flow Measurement Complete"=w232:bool, "Vacuum Data"=w256:dbl)  [unwired: 1 in, 2 out]
            "Pressure Decay Hold Test Complete" <- w232
            "STOP Button Pressed 4" <- w260
            n66 = Unbundle By Name(w237) -> ("Press Decay Ref"=w231:refnum<vi>, "Table Control"=w234:refnum<vi>, "Table Control"=w238:string[][], "Max Vacuum"=w233:dbl)
            n67 = Subtract(x=w233, y=w256) -> (x-y=w255:dbl)
            n68 = call "TestStatusTableBuilder.vi"("array"=w238, "Test Case Timeout"=FALSE, "STOP Button Pressed"=w260, "Test Case Target Reached"=w232, "Test State"="Pressure Decay Monitoring", "Test Status"="Decay Data Collected", "Measurement"=w255, "Units"="PSI") -> ("Table Control"=w235:string[][])  [unwired: 7 in]
            n69 = property class="Bool (strict)"(reference=w231, "Value"=w232) -> ()  [unwired: 1 in, 2 out]
            n70 = property class="Tbl (strict)"(reference=w234, "Value"=w235) -> ()  [unwired: 1 in, 2 out]
            n71 = Bundle By Name(cluster=w237, "Table Control"=w235) -> (w236:T5)
            n72 = call-poly "Enqueue Message.vi"("error in (no error)"=w241, "Message"="Manual Acquire", "Message Queue"=w243) -> ("error out"=w244:errorcluster)  [unwired: 7 in, 1 out]
            n73 = call-poly "Enqueue Message.vi"("error in (no error)"=w241, "Message Data"="Benchmarking Complete. Data Saved to File." ("Message"), "Message"="Update Status", "Message Queue"=w242) -> ("error out"=w246:errorcluster, "dup Message Queue"=w247:refnum<queue>)  [unwired: 6 in]
            n74 = call-poly "Enqueue Message.vi"("error in (no error)"=w246, "Message"="Init Valves", "Message Queue"=w247) -> ()  [unwired: 7 in, 2 out]
          }
          frame "Stop" {
            # "Stop - Stop the Acquisition. Also flush the queue of any pending \"Acquire\" messages."
            n75 = case shown="\"Acquiring\"" w274 {
              selector: w274 -> [w280 _]
              tunnel: w277 -> [w279 w289]
              tunnel: w269 -> [_ w288]
              tunnel: w276 -> [_ w286]
              tunnel: w275 -> [_ w285]
              tunnel: [w280 Acquisition_State."Idle" ("State")] -> w273
              tunnel: [w279 w283] -> w272
              frame "Idle", Default {
                # "The system is already idle. Ignore the \"Stop\" message."
              }
              frame "Acquiring" {
                # "If the system is acquiring, stop the acquisition."
                n76 = Flush Queue(queue=w286, error in (no error)=w289) -> (error out=w287:errorcluster)  [unwired: 2 out]
                n77 = call "Stop Acquisition.vi"("error in (no error)"=w287, "Hardware Resources in"=w288) -> ("error out"=w284:errorcluster)  [unwired: 9 in]
                n78 = call-poly "Enqueue Message.vi"("error in (no error)"=w284, "Message"="Acquisition Stopped", "Message Queue"=w285) -> ("error out"=w283:errorcluster)  [unwired: 7 in, 1 out]
              }
            }
            n79 = Merge Errors(w272) -> (w278:errorcluster)
            n80 = Bundle By Name(cluster=w269, "Cycle Count"=u64 0) -> (w268:T5)
          }
          frame "Exit" {
            # "Don't check the error out. The UI message queue may have already been released."
            # "Release the Acquisition queue reference"
            # "Stop the VI"
            # "Exit - Send the Exit message to the UI Message Handler."
            n81 = Release Queue(queue=w293, error in (no error)=w297) -> (error out=w294:errorcluster)  [unwired: 1 in, 2 out]
            n82 = call "Stop Acquisition.vi"("Hardware Resources in"=w292) -> ()  [unwired: 10 in, 1 out]
            n83 = call-poly "Enqueue Message.vi"("Priority Message? (F)"=TRUE, "Message"="Exit", "Message Queue"=w298) -> ()  [unwired: 7 in, 2 out]
            n84 = Merge Errors(w294) -> (w299:errorcluster)
          }
          frame Default {
            # "'Default' case only runs if there is a message that isn't defined in any of the other cases.  Output a programming error."
            n85 = xnode "Error Ring"("parameter 0"=w304) -> ("error out"=w303:errorcluster)
          }
        }
        n86 = call "Error Handler - Acquisition Message Loop.vi"("error in (no error)"=w29, "Message Queue"=w27) -> ("dup error in"=w28:errorcluster)  [unwired: 8 in, 1 out]
      }
    }
    frame Error {
    }
  }
  "error out" <- w5
  n87 = disable-structure shown="Disabled" {
    disable-tunnel: _ -> [w314 _]
    frame Disabled {
      w322 = T6 {"Row"=0, "Column"=0} ("Selection Size")
      n88 = Unbundle By Name(w314) -> ("TestConfigDisplay"=w315)
      n89 = feedback #1(1 ("Row")) -> (w317:i32)
      n90 = Increment(x=w317) -> (x+1=w316:i32)
      n91 = feedback-in #1(w316) -> ()
      n92 = Bundle By Name(cluster=w322, "Row"=1, "Column"=9) -> (w323:T6)
      n93 = Bundle By Name(cluster=w322, "Row"=w316) -> (w321:T6)
      n94 = property class="Tbl (strict)"(reference=w315, "Selection Size"=w323, "Selection Start"=w321) -> ()  [unwired: 1 in, 2 out]
    }
    frame Enabled {
    }
  }
